vi "End.vi"(8 "error in (no error)":errorcluster, 11 "Channel in":refnum<class "Channel.lvclass">) -> (0 "error out":errorcluster, 3 "Channel out":refnum<class "Channel.lvclass">)   [LabVIEW 2018, in "Channel.lvclass"]
doc: "End the ACS execution \n\nThis function is responsible for eding the ACS execution correctly"
uses:
  Channel.lvclass
  Channel.lvclass/Channel.ctl
  RxTx/RxTx.lvclass
  Simulated_CCD_Camera/Simulated_CCD_Camera.lvclass
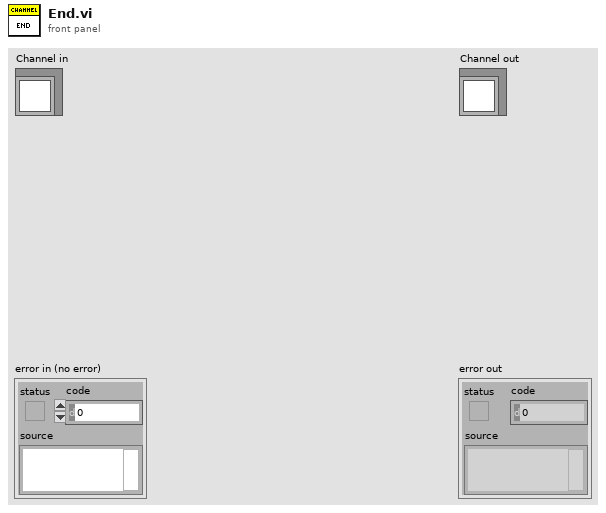
[diagram p1: front panel]
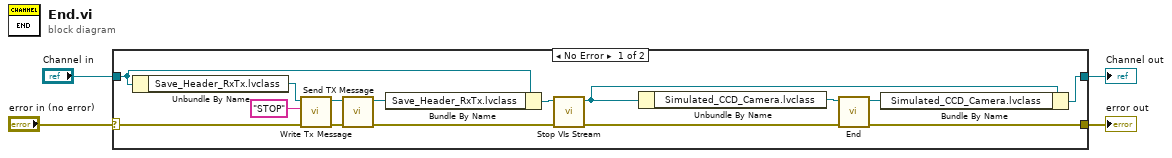
[diagram p0: block diagram]
diagram:
  n1 = case shown="No Error" "error in (no error)" {
    selector: "error in (no error)" -> [w8 w21]
    tunnel: [w12 w21] -> w3
    tunnel: [w15 w20] -> w1
    tunnel: "Channel in" -> [w19 w20]
    frame No Error {
      n2 = Unbundle By Name(w19) -> ("Save_Header_RxTx.lvclass"=w11:refnum<class "RxTx.lvclass">)
      n3 = call "Write Tx Message.vi"("error in (no error)"=w8, "Tx Message"="STOP" ("element"), "RxTx in"=w11) -> ("error out"=w9:errorcluster, "RxTx out"=w10:refnum<class "RxTx.lvclass">)  [unwired: 7 in]
      n4 = call "Send TX Message.vi"("error in (no error)"=w9, "RxTx in"=w10) -> ("error out"=w16:errorcluster, "RxTx out"=w17:refnum<class "RxTx.lvclass">)  [unwired: 8 in]
      n5 = Bundle By Name(cluster=w19, "Save_Header_RxTx.lvclass"=w17) -> (w18:refnum<class "Channel.lvclass">)
      n6 = call "Stop VIs Stream.vi"("error in (no error)"=w16, "Channel in"=w18) -> ("error out"=w5:errorcluster, "Channel out"=w6:refnum<class "Channel.lvclass">)  [unwired: 8 in]
      n7 = Unbundle By Name(w6) -> ("Simulated_CCD_Camera.lvclass"=w14:refnum<class "Simulated_CCD_Camera.lvclass">)
      n8 = call "End.vi"("error in (no error)"=w5, "Simulated_CCD_Camera in"=w14) -> ("error out"=w12:errorcluster, "Simulated_CCD_Camera out"=w13:refnum<class "Simulated_CCD_Camera.lvclass">)  [unwired: 8 in]
      n9 = Bundle By Name(cluster=w6, "Simulated_CCD_Camera.lvclass"=w13) -> (w15:refnum<class "Channel.lvclass">)
    }
    frame Error {
    }
  }
  "error out" <- w3
  "Channel out" <- w1
